vi "Get Library Name.vi"(11 "LVLIBP Parser in":refnum<class "LVLIBP Parser.lvclass">) -> (2 "Library Name":string, 3 "LVLIBP Parser out":refnum<class "LVLIBP Parser.lvclass">)   [LabVIEW 2019, in "LVLIBP CD XML Updater.lvlib" / "LVLIBP Parser.lvclass"]
uses:
  LVLIBP Parser.lvclass
  LVLIBP Parser.lvclass/LVLIBP Parser.ctl
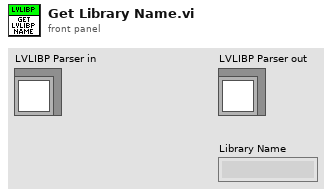
[diagram p1: front panel]
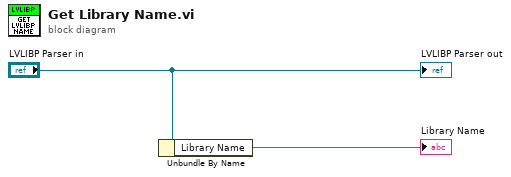
[diagram p0: block diagram]
diagram:
  n1 = Unbundle By Name("LVLIBP Parser in") -> ("Library Name"=→"Library Name":string)
  "LVLIBP Parser out" <- "LVLIBP Parser in"
